vi "LuaVIEW Error Handling.vi"() -> (0 "pass?":bool)   [LabVIEW 2012]
panel:
  in  "test script":string="success,errormsg = lv.pcall(do_script,\"test 1\",[[\n]])\nif (not success) then error(\"Empty scripts should not fail\") end\n\nsuccess,errormsg = lv.pcall(do_script,\"test 2\",[[\nerror(\"Some Lua error\")\n]])\nif (success) then error(\"Expected to catch a Lua error\") end\n\nsuccess,errormsg = lv.pcall(do_script,\"test 3\",[[\nmsg.send(\"nonexistingtask\",\"some message\")\n]])\nif (success) then error(\"Expected to catch a LabVIEW error\") end\n\nsuccess,errormsg = lv.pcall(do_script,\"test 4\",[[\npcall(error, \"Some Lua error\")\n]])\nif (not success) then error(\"pcall() should catch Lua errors\") end\n"
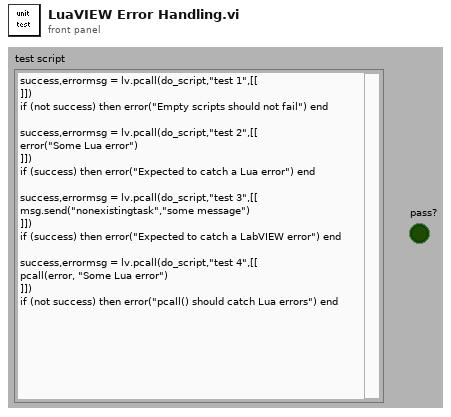
[diagram p1: front panel]
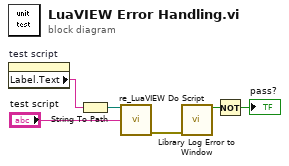
[diagram p0: block diagram]
diagram:
  n1 = property on="test script" class="Str"() -> ("Label.Text"=w2:string)  [unwired: 2 in, 2 out]
  n2 = String To Path(string=w2) -> (path=w1:path)
  n3 = call "re_LuaVIEW Do Script.vi"("script file or name (no name)"=w1, "script string (\"\" == load from file)"="test script") -> ("error out"=w4:errorcluster)  [unwired: 13 in]
  n4 = call "Library Log Error to Window.vi"("error in (no error)"=w4) -> ("error?"=w6:bool)  [unwired: 13 in, 1 out]
  n5 = Not(x=w6) -> (.not. x?=→"pass?":bool)
